vi "match_dsp_serialvi.vi"() -> ()   [LabVIEW 2024]
uses:
  <vilib>/Instr/_visa.llb/VISA Configure Serial Port (Instr).vi
panel:
  in  "?":i32 min=0 max=5 step=1
  in  "?":i32 min=0 max=4000 step=1
  in  "?":i32=10 min=10 max=1600 step=10
  out "?":i32
  out "?":bool
  out "?":dbl
  in  "?":u32=1 min=1 max=4 step=1
  out "command response":string
  out "command send":string
  out "Power":bool
  out "Ready":bool
  in  "Write Function Generator Waveform":bool
  in  "Write Function Generator Amplitude":bool
  in  "Write Function Generator Frequency":bool
  in  "Activate Current Tuning Number":bool
  in  "Read Tunning Number":bool
  in  "Read Power Supply Voltage Levels":bool
  in  "Servo Status Flags":bool
  in  "?":bool
  in  "COM":refnum<visa-resource-name>
  # "X- axis"
  # "(+) volts"
  # "Command Sent"
  # "Command Response"
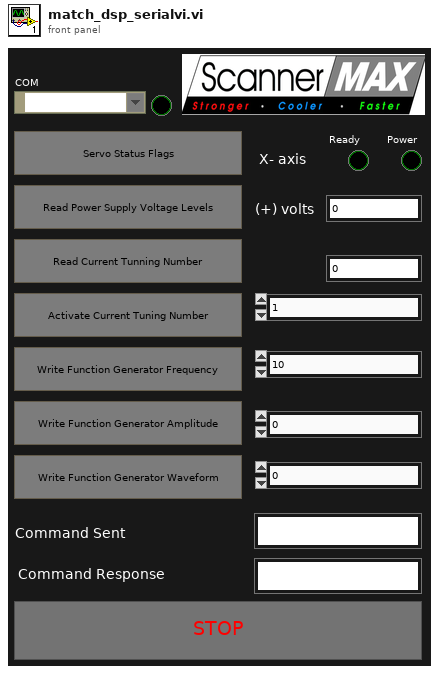
[diagram p1: front panel]
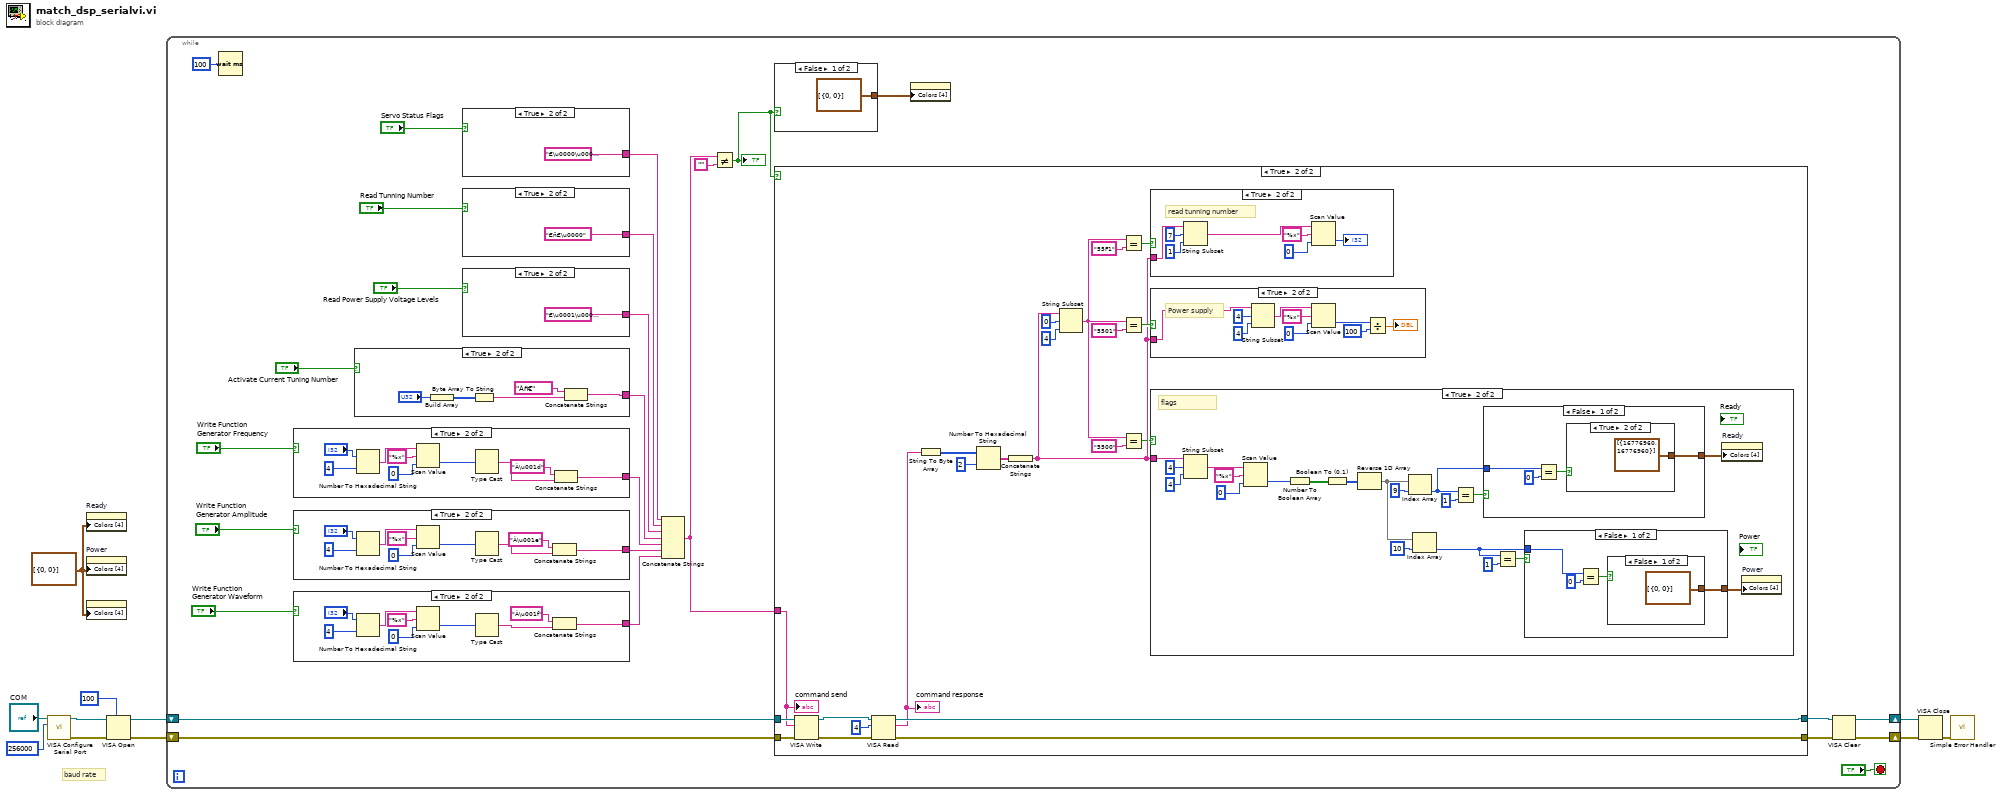
[diagram p0: block diagram]
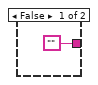
[diagram p2: hidden frame]
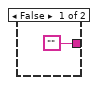
[diagram p3: hidden frame]
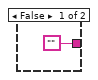
[diagram p4: hidden frame]
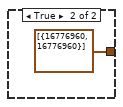
[diagram p5: hidden frame]
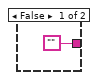
[diagram p6: hidden frame]
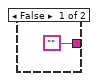
[diagram p7: hidden frame]
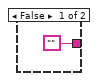
[diagram p8: hidden frame]
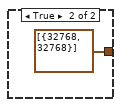
[diagram p11: hidden frame]
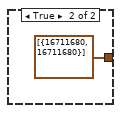
[diagram p12: hidden frame]
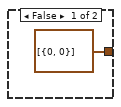
[diagram p13: hidden frame]
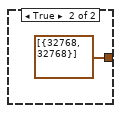
[diagram p14: hidden frame]
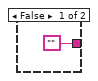
[diagram p17: hidden frame]
diagram:
  w1 = cluster{u32, u32}[] [{0, 0}] ("Colors [4]")
  # "baud rate"
  n1 = call-poly "VISA Configure Serial Port"("VISA resource name"="COM", "baud rate (9600)"=u32 256000) -> ("VISA resource name out"=w11:refnum<visa-resource-name>, "error out"=w8:errorcluster)  [unwired: 12 in]
  n2 = property on="Ready" class="Bool (strict)"("Colors [4]"=w1) -> ()  [unwired: 2 in, 2 out]
  n3 = property on="Power" class="Bool (strict)"("Colors [4]"=w1) -> ()  [unwired: 2 in, 2 out]
  n4 = property class="Bool (strict)"("Colors [4]"=w1) -> ()  [unwired: 2 in, 2 out]
  n5 = VISA Open(timeout (0)=u32 100 ("VISA Open timeout (0)"), error in (no error)=w8, VISA resource name=w11) -> (VISA resource name=w7:refnum<visa-resource-name>, error out=w6:errorcluster)  [unwired: 2 in]
  n6 = while {
    shift-right: [w34] -> w5
    shift-left: w7 -> [w36]
    shift-right: [w33] -> w4
    shift-left: w6 -> [w35]
    stop <- "?" stop-if-true
    n7 = Wait (ms)(milliseconds to wait=u32 100) -> ()  [unwired: 1 out]
    n8 = case shown="True" "Write Function Generator Frequency" {
      tunnel: ["" w64] -> w16
      frame False {
      }
      frame True {
        n9 = Number To Hexadecimal String(1:i16 4 ("width (-)"), 2:"?") -> (0:w61:string)
        n10 = Scan Value(string=w61, format string="%x", default (0 dbl)=i16 0) -> (value=w60:i16)  [unwired: 1 out]
        n11 = Type Cast(x=w60) -> (*(type *) &x=w59:string)  [unwired: 1 in]
        n12 = Concatenate Strings("À\u001d", w59) -> (w64:string)
      }
    }
    n13 = case shown="True" "Write Function Generator Amplitude" {
      tunnel: ["" w54] -> w14
      frame False {
      }
      frame True {
        n14 = Number To Hexadecimal String(1:i16 4 ("width (-)"), 2:"?") -> (0:w51:string)
        n15 = Scan Value(string=w51, format string="%x", default (0 dbl)=i16 0) -> (value=w50:i16)  [unwired: 1 out]
        n16 = Type Cast(x=w50) -> (*(type *) &x=w49:string)  [unwired: 1 in]
        n17 = Concatenate Strings("À\u001e", w49) -> (w54:string)
      }
    }
    n18 = case shown="True" "Write Function Generator Waveform" {
      tunnel: ["" w44] -> w12
      frame False {
      }
      frame True {
        n19 = Number To Hexadecimal String(1:i16 4 ("width (-)"), 2:"?") -> (0:w41:string)
        n20 = Scan Value(string=w41, format string="%x", default (0 dbl)=i16 0) -> (value=w40:i16)  [unwired: 1 out]
        n21 = Type Cast(x=w40) -> (*(type *) &x=w39:string)  [unwired: 1 in]
        n22 = Concatenate Strings("À\u001f", w39) -> (w44:string)
      }
    }
    n23 = case shown="True" "Activate Current Tuning Number" {
      tunnel: ["" w74] -> w20
      frame False {
      }
      frame True {
        n24 = Build Array("?") -> (w72:u32[])
        n25 = Byte Array To String(unsigned byte array=w72) -> (string=w71:string)
        n26 = Concatenate Strings("Àñ€", w71) -> (w74:string)
      }
    }
    n27 = case shown="True" "Servo Status Flags" {
      tunnel: ["" "€\u0000\u0000\u0000"] -> w26
      frame False {
      }
      frame True {
      }
    }
    n28 = case shown="True" "Read Tunning Number" {
      tunnel: ["" "€ñ€\u0000"] -> w25
      frame False {
      }
      frame True {
      }
    }
    n29 = case shown="True" "Read Power Supply Voltage Levels" {
      tunnel: ["" "€\u0001\u0000\u0000"] -> w22
      frame False {
      }
      frame True {
      }
    }
    n30 = Concatenate Strings(w26, w25, w22, w20, w16, w14, w12) -> (w24:string)
    n31 = Not Equal?(x=w24, y="") -> (x != y?=w19:bool)
    "?" <- w19
    n32 = case shown="False" w19 {
      tunnel: [cluster{u32, u32}[] [{0, 0}] ("Colors [4]") cluster{u32, u32}[] [{16776960, 16776960}] ("Colors [4]")] -> w18
      frame False {
      }
      frame True {
      }
    }
    n33 = case shown="True" w19 {
      tunnel: w24 -> [_ w97]
      tunnel: w36 -> [w81 w100]
      tunnel: w35 -> [w80 w99]
      tunnel: [w81 w98] -> w29
      tunnel: [w80 w96] -> w28
      frame False {
      }
      frame True {
        n34 = VISA Write(VISA resource name=w100, write buffer=w97, error in (no error)=w99) -> (VISA resource name out=w102:refnum<visa-resource-name>, error out=w103:errorcluster)  [unwired: 1 out]
        n35 = VISA Read(VISA resource name=w102, byte count=u32 4, error in (no error)=w103) -> (VISA resource name out=w98:refnum<visa-resource-name>, read buffer=w94:string, error out=w96:errorcluster)  [unwired: 1 out]
        "command response" <- w94
        n36 = String To Byte Array(string=w94) -> (unsigned byte array=w92:u8[])
        n37 = Number To Hexadecimal String(1:i16 2 ("width (-)"), 2:w92) -> (0:w95:string[])
        n38 = Concatenate Strings(w95) -> (w85:string)
        n39 = String Subset(string=w85, offset (0)=0, length (rest)=4 ("length (rest)")) -> (substring=w82:string)
        n40 = Equal?(x=w82, y="55F1") -> (x = y?=w86:bool)
        n41 = Equal?(x=w82, y="5501") -> (x = y?=w90:bool)
        n42 = Equal?(x=w82, y="5500") -> (x = y?=w83:bool)
        n43 = case shown="True" w86 {
          tunnel: w85 -> [_ w139]
          frame False {
          }
          frame True {
            # "read tunning number"
            n44 = String Subset(string=w139, offset (0)=7, length (rest)=1 ("length (rest)")) -> (substring=w138:string)
            n45 = Scan Value(string=w138, format string="%x", default (0 dbl)=0) -> (value=→"?":i32)  [unwired: 1 out]
          }
        }
        n46 = case shown="True" w90 {
          tunnel: w85 -> [_ w146]
          frame False {
          }
          frame True {
            # "Power supply"
            n47 = String Subset(string=w146, offset (0)=4, length (rest)=4 ("length (rest)")) -> (substring=w145:string)
            n48 = Scan Value(string=w145, format string="%x", default (0 dbl)=0) -> (value=w151:i32)  [unwired: 1 out]
            n49 = Divide(x=w151, y=100) -> (x/y=→"?":dbl)
          }
        }
        n50 = case shown="True" w83 {
          tunnel: w85 -> [_ w119]
          frame False {
          }
          frame True {
            # "flags"
            n51 = String Subset(string=w119, offset (0)=4, length (rest)=4 ("length (rest)")) -> (substring=w114:string)
            n52 = Scan Value(string=w114, format string="%x", default (0 dbl)=i16 0) -> (value=w118:i16)  [unwired: 1 out]
            n53 = Number To Boolean Array(number=w118) -> (Boolean array=w117:bool[])
            n54 = Boolean To (0,1)(Boolean=w117) -> (0, 1=w116:i16[])
            n55 = Reverse 1D Array(array=w116) -> (reversed array=w112:i16[])
            n56 = Index Array(array=w112, index=9) -> (element=w108:i16)
            n57 = Index Array(array=w112, index=10) -> (element=w104:i16)
            n58 = Equal?(x=w108, y=i16 1) -> (x = y?=w111:bool)
            n59 = case shown="False" w111 {
              tunnel: [w131 cluster{u32, u32}[] [{32768, 32768}] ("Colors [4]")] -> w109
              tunnel: w108 -> [w134 _]
              frame False {
                n60 = Equal?(x=w134, y=i16 0) -> (x = y?=w132:bool)
                n61 = case shown="True" w132 {
                  tunnel: [cluster{u32, u32}[] [{0, 0}] ("Colors [4]") cluster{u32, u32}[] [{16776960, 16776960}] ("Colors [4]")] -> w131
                  frame False {
                  }
                  frame True {
                  }
                }
              }
              frame True {
              }
            }
            n62 = Equal?(x=w104, y=i16 1) -> (x = y?=w106:bool)
            n63 = case shown="False" w106 {
              tunnel: [w124 cluster{u32, u32}[] [{16711680, 16711680}] ("Colors [4]")] -> w105
              tunnel: w104 -> [w127 _]
              frame False {
                n64 = Equal?(x=w127, y=i16 0) -> (x = y?=w125:bool)
                n65 = case shown="False" w125 {
                  tunnel: [cluster{u32, u32}[] [{0, 0}] ("Colors [4]") cluster{u32, u32}[] [{32768, 32768}] ("Colors [4]")] -> w124
                  frame False {
                  }
                  frame True {
                  }
                }
              }
              frame True {
              }
            }
            n66 = property on="Ready" class="Bool (strict)"("Colors [4]"=w109) -> ()  [unwired: 2 in, 2 out]
            n67 = property on="Power" class="Bool (strict)"("Colors [4]"=w105) -> ()  [unwired: 2 in, 2 out]
          }
        }
        "command send" <- w97
      }
    }
    n68 = property class="Bool (strict)"("Colors [4]"=w18) -> ()  [unwired: 2 in, 2 out]
    n69 = VISA Clear(VISA resource name=w29, error in (no error)=w28) -> (VISA resource name out=w34:refnum<visa-resource-name>, error out=w33:errorcluster)
  }
  n70 = VISA Close(VISA resource name=w5, error in (no error)=w4) -> (error out=w2:errorcluster)
  n71 = call <vilib>:"Simple Error Handler.vi"("error in (no error)"=w2) -> ()  [unwired: 4 in, 5 out]
